vi "SubVI_Izhikevich_001.vi"(1 "I":dbl(slide) scale=0.0..10.0, 2 "Neuron Model Selector":T1(ring)) -> (0 "v":dbl(graph))   [LabVIEW 2018]
panel:
  in  "stop":bool
  out "u":dbl(graph)
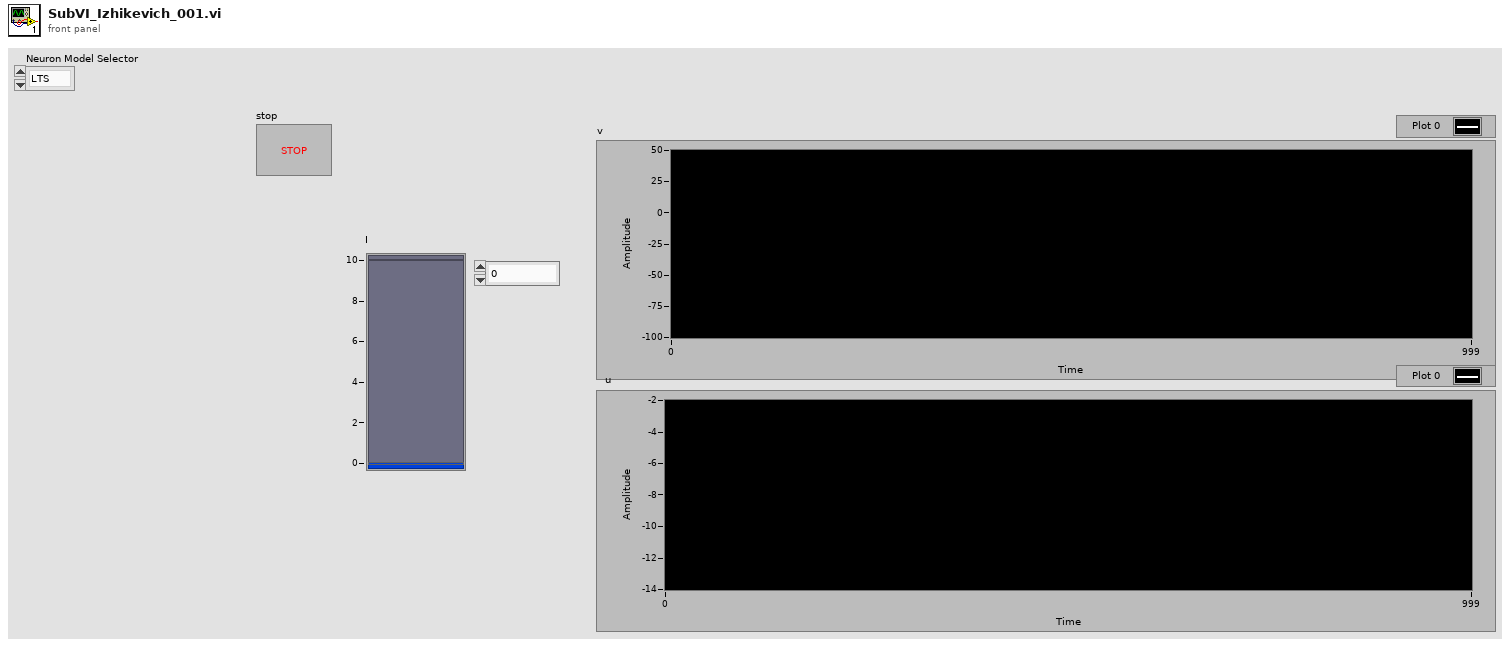
[diagram p1: front panel]
types:
  T1 = enum16{"LTS", "RZ", "TC2", "TC1", "FS", "CH", "IB", "RS"}
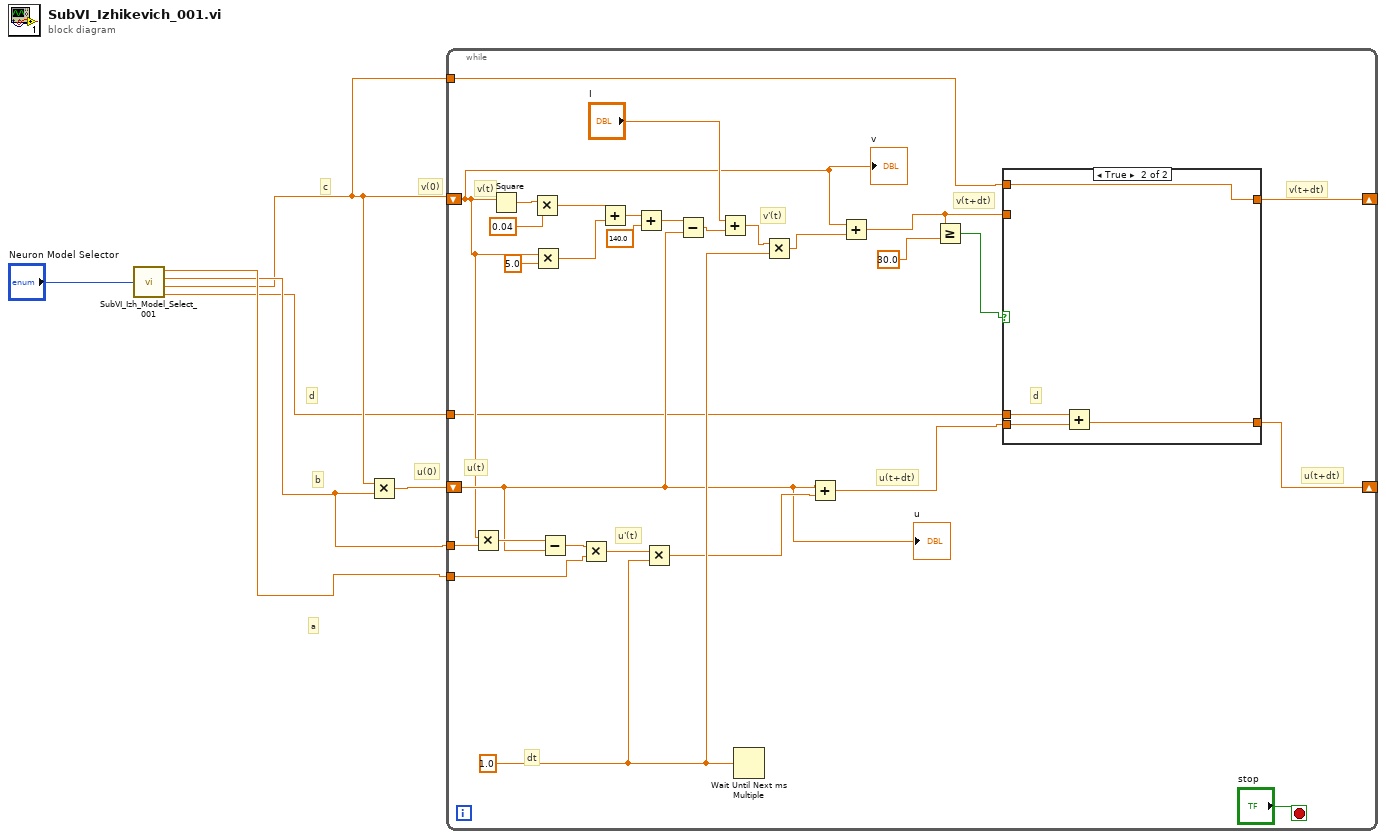
[diagram p0: block diagram]
diagram:
  # "d"
  # "a"
  # "u(0)"
  # "v(0)"
  # "c"
  # "b"
  n1 = call "SubVI_Izh_Model_Select_001.vi"("Neuron Model Selector"="Neuron Model Selector") -> ("a"=w5:dbl, "b"=w4:dbl, "c"=w3:dbl, "d"=w2:dbl)
  n2 = Multiply(x=w3, y=w4) -> (x*y=w6:dbl)
  n3 = while {
    shift-right: [w13] -> _
    shift-left: w3 -> [w8]
    shift-right: [w15] -> _
    shift-left: w6 -> [w10]
    tunnel: w4 -> [w24]
    tunnel: w5 -> [w21]
    tunnel: w3 -> [w12]
    tunnel: w2 -> [w7]
    stop <- "stop" stop-if-true
    w19 = 1.0 ("millisecond multiple")
    # "u(t+dt)"
    # "u(t+dt)"
    # "v(t+dt)"
    # "u'(t)"
    # "v'(t)"
    # "dt"
    # "v(t+dt)"
    # "u(t)"
    # "v(t)"
    n4 = Multiply(x=w8, y=w24) -> (x*y=w23:dbl)
    n5 = Square(x=w8) -> (x^2=w36:dbl)
    n6 = Multiply(x=w36, y=0.04) -> (x*y=w32:dbl)
    n7 = Multiply(x=w8, y=5.0) -> (x*y=w33:dbl)
    n8 = Subtract(x=w23, y=w10) -> (x-y=w22:dbl)
    n9 = Multiply(x=w22, y=w21) -> (x*y=w20:dbl)
    n10 = Add(x=w32, y=w33) -> (x+y=w31:dbl)
    n11 = Add(x=w31, y=140.0) -> (x+y=w29:dbl)
    n12 = Multiply(x=w20, y=w19) -> (x*y=w18:dbl)
    n13 = Subtract(x=w29, y=w10) -> (x-y=w27:dbl)
    n14 = Add(x="I", y=w27) -> (x+y=w28:dbl)
    n15 = Wait Until Next ms Multiple(millisecond multiple=w19) -> ()  [unwired: 1 out]
    n16 = Multiply(x=w28, y=w19) -> (x*y=w25:dbl)
    n17 = Add(x=w10, y=w18) -> (x+y=w9:dbl)
    n18 = Add(x=w8, y=w25) -> (x+y=w14:dbl)
    n19 = Greater Or Equal?(x=w14, y=30.0) -> (x >= y?=w16:bool)
    n20 = case shown="True" w16 {
      tunnel: w9 -> [w38 w41]
      tunnel: [w38 w40] -> w15
      tunnel: w14 -> [w37 _]
      tunnel: [w37 w42] -> w13
      tunnel: w12 -> [_ w42]
      tunnel: w7 -> [_ w39]
      frame False {
      }
      frame True {
        # "d"
        n21 = Add(x=w39, y=w41) -> (x+y=w40:dbl)
      }
    }
    "v" <- w8
    "u" <- w10
  }
